vi "Initialize Lights.vi"(8 "error in (no error)":errorcluster, 11 "Controls[]":refnum<vi>[](array[refnum])) -> (0 "error out":errorcluster)   [LabVIEW 2016]
doc: "Initialize Zone Status indicators to their defaults."
uses:
  Controls/Zones Condition.ctl
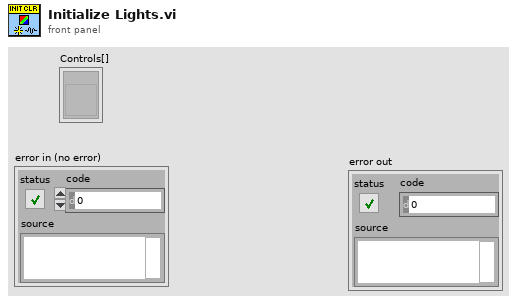
[diagram p1: front panel]
types:
  T1 = typedef "Zones Condition.ctl" = enum16{"Normal", "Bypass", "Tamper", "Alarm"}
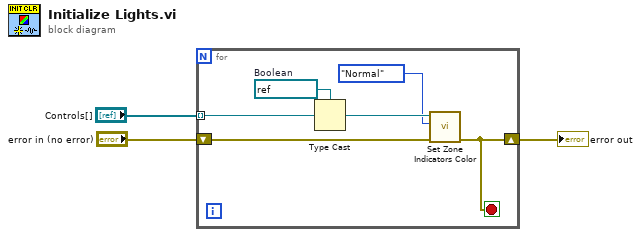
[diagram p0: block diagram]
diagram:
  n1 = for {
    tunnel: "Controls[]" -> [w8] mode=indexing
    shift-right: [w4] -> w3
    shift-left: "error in (no error)" -> [w5]
    stop <- w4 stop-if-true
    w9 = refnum<vi> refnum  # Boolean
    n2 = Type Cast(type=w9, x=w8) -> (*(type *) &x=w7:refnum<vi>)
    n3 = call "Set Zone Indicators Color.vi"("error in"=w5, "Alert Status"=Zones_Condition."Normal", "reference"=w7) -> ("error out"=w4:errorcluster)  [unwired: 8 in]
  }
  "error out" <- w3
